vi "Module_Template.vi"(11 "Cluster":T2) -> ()   [LabVIEW 2014]
uses:
  User_Event/TypeDef.ctl
  Control/Queue_Message_TypeDef.ctl
  QSM/TypeDef.ctl
  <vilib>/Utility/error.llb/Error Cluster From Error Code.vi
  <vilib>/ErrorRing/Error Ring.xnode
  QSM/Queue_Library.lvlib
  User_Event/User_Event_Library.lvlib
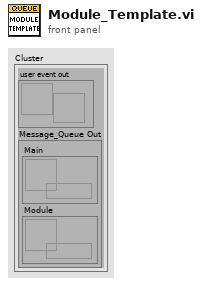
[diagram p1: front panel]
types:
  T1 = typedef "Queue_Message_TypeDef.ctl" = cluster{"Main":refnum<queue>, "Module":refnum<queue>}
  T2 = cluster{"user event out":refnum<user-event>, "Message_Queue Out":T1}
  T3 = cluster{"Number":i32, "Variant":variant, "ST":string, "ST_array":string[], "Number_Array":i32[]}
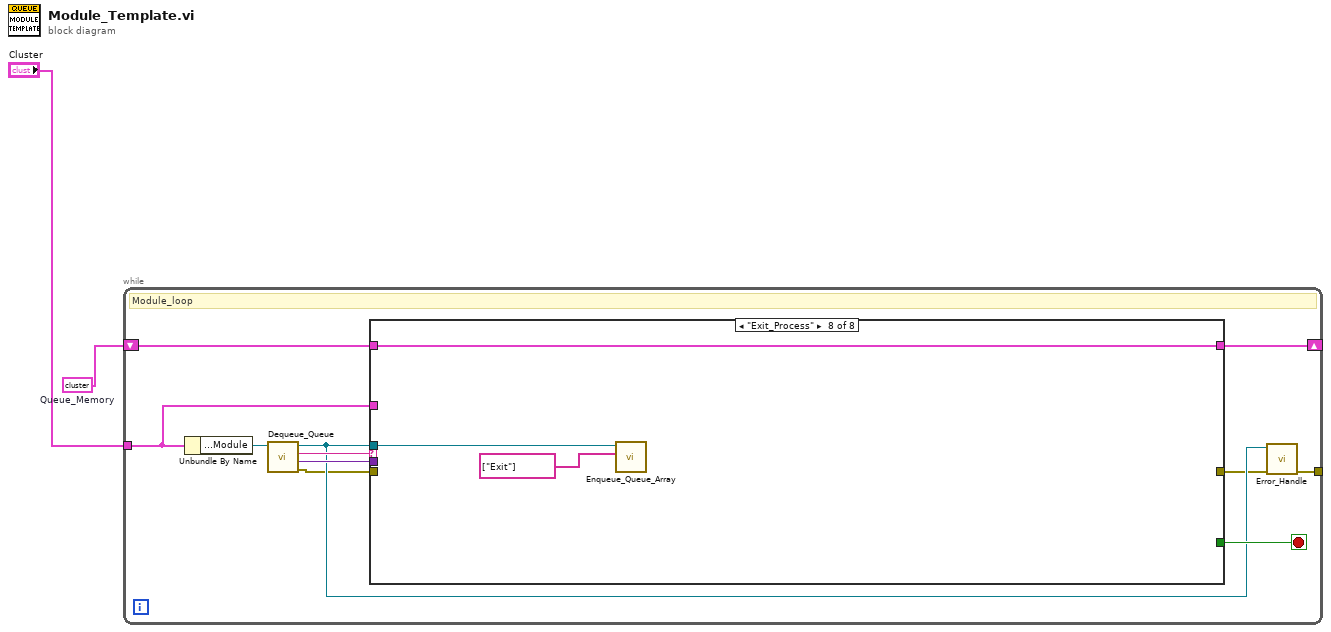
[diagram p0: block diagram]
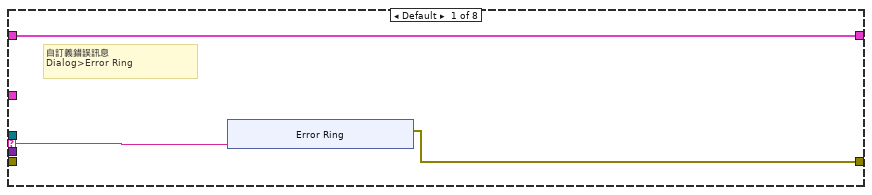
[diagram p2: hidden frame]
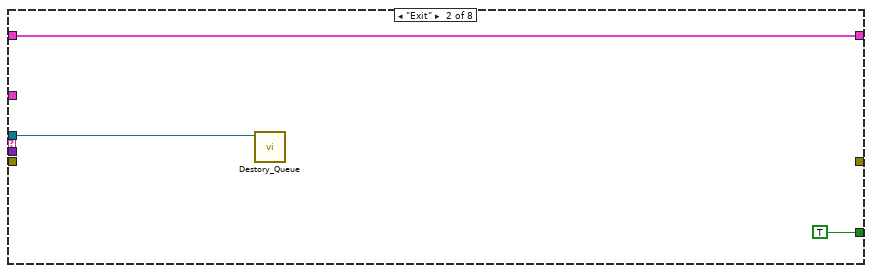
[diagram p3: hidden frame]
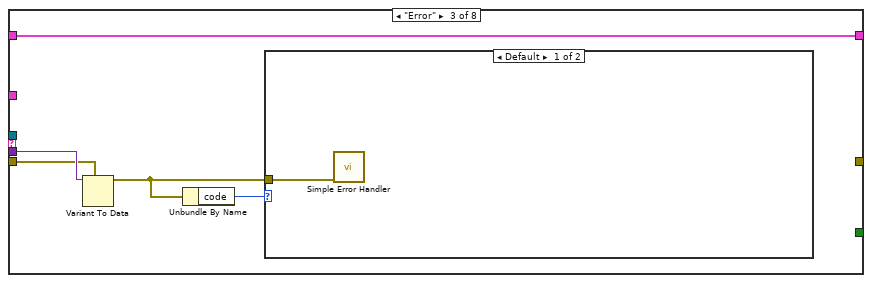
[diagram p4: hidden frame]
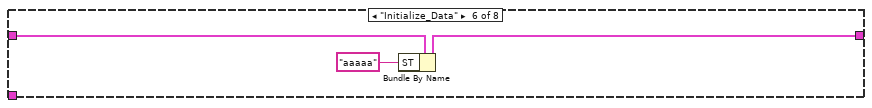
[diagram p8: hidden frame]
diagram:
  w2 = T3 {"Number"=0, "Variant"=variant, "ST"="", "ST_array"=[], "Number_Array"=[]}  # Queue_Memory
  n1 = while {
    tunnel: "Cluster" -> [w9]
    shift-right: [w8] -> _
    shift-left: w2 -> [w7]
    tunnel: [w3] -> _
    stop <- w12 stop-if-true
    # "Module_loop"
    n2 = Unbundle By Name(w9) -> ("Message_Queue Out.Module"=w10:refnum<queue>)
    n3 = call "Dequeue_Queue.vi"("queue In"=w10) -> ("error out"=w4:errorcluster, "Data"=w11:variant, "Command"=w13:string, "queue Out"=w6:refnum<queue>)  [unwired: 7 in]
    n4 = case shown="\"Exit_Process\"" w13 {
      selector: w13 -> [w14 _ _ _ _ _ _ _]
      tunnel: w6 -> [_ w24 _ _ _ _ _ w43]
      tunnel: [_ TRUE _ _ _ _ _ _] -> w12
      tunnel: w11 -> [_ _ w30 _ _ _ _ _]
      tunnel: w9 -> [_ _ _ _ _ _ _ _]
      tunnel: [w16 w25 w31 w33 w35 w37 w40 w41] -> w8
      tunnel: w7 -> [w16 w25 w31 w33 w35 w38 w40 w41]
      tunnel: [w15 _ _ _ w34 _ w39 _] -> w5
      tunnel: w4 -> [_ _ w29 _ w34 _ w39 _]
      frame Default {
        # "自訂義錯誤訊息\nDialog>Error Ring"
        n5 = xnode "Error Ring"("parameter 0"=w14) -> ("error out"=w15:errorcluster)
      }
      frame "Exit" {
        n6 = call "Destory_Queue.vi"("queue In"=w24) -> ()  [unwired: 10 in, 1 out]
      }
      frame "Error" {
        n7 = Variant To Data(type=w29, Variant=w30) -> (data=w27:errorcluster)  [unwired: 1 in, 1 out]
        n8 = Unbundle By Name(w27) -> ("code"=w28:i32)
        n9 = case shown="Default" w28 {
          tunnel: w27 -> [w32 _]
          frame Default {
            n10 = call <vilib>:"Simple Error Handler.vi"("error in (no error)"=w32) -> ()  [unwired: 4 in, 5 out]
          }
          frame 56 {
          }
        }
      }
      frame "------Initialize------" {
      }
      frame "Initialize" {
      }
      frame "Initialize_Data" {
        n11 = Bundle By Name(cluster=w38, "ST"="aaaaa") -> (w37:T3)
      }
      frame "------Function------" {
      }
      frame "Exit_Process" {
        n12 = call "Enqueue_Queue_Array.vi"("Command"=string[] ["Exit"], "queue In"=w43) -> ()  [unwired: 8 in, 2 out]
      }
    }
    n13 = call "Error_Handle.vi"("error in (no error)"=w5, "queue In"=w6) -> ("error out"=w3:errorcluster)  [unwired: 8 in, 1 out]
  }
